vi "Passive Torque Calculator.vi"(11 "Sensors":T1) -> (2 "Passive Torque Estimate":dbl)   [LabVIEW 2018]
uses:
  Sensor Data.ctl
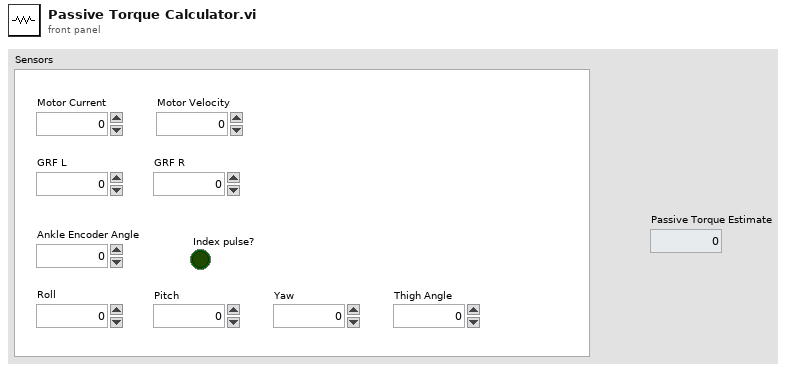
[diagram p1: front panel]
types:
  T1 = typedef "Sensor Data.ctl" = cluster{"Motor Current":dbl, "Motor Velocity":dbl, "Ankle Encoder Angle":dbl, "GRF L":dbl, "GRF R":dbl, "Index pulse?":bool, "Roll":dbl, "Pitch":dbl, "Yaw":dbl, "Thigh Angle":dbl}
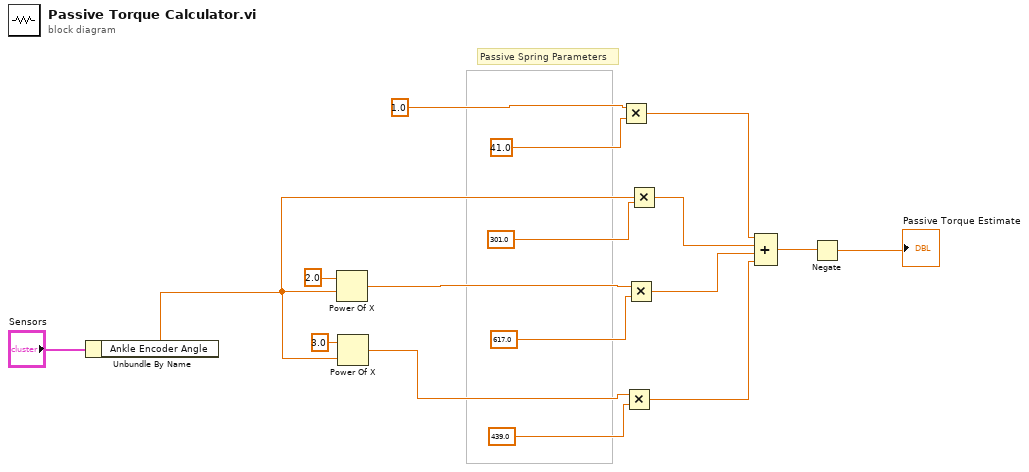
[diagram p0: block diagram]
diagram:
  # "Passive Spring Parameters"
  n1 = Unbundle By Name("Sensors") -> ("Ankle Encoder Angle"=w10:dbl)
  n2 = Power Of X(1:w10, 2:2.0 ("y")) -> (0:w11:dbl)
  n3 = Power Of X(1:w10, 2:3.0 ("y")) -> (0:w13:dbl)
  n4 = Multiply(x=1.0, y=41.0) -> (x*y=w6:dbl)
  n5 = Multiply(x=w13, y=439.0) -> (x*y=w3:dbl)
  n6 = Multiply(x=w11, y=617.0) -> (x*y=w4:dbl)
  n7 = Multiply(x=w10, y=301.0) -> (x*y=w5:dbl)
  n8 = Compound Arithmetic op=ADD(w6, w5, w4, w3) -> (w2:dbl)
  n9 = Negate(x=w2) -> (-x=→"Passive Torque Estimate":dbl)
